vi "2진파일 읽기_쓰기.vi"() -> ()   [LabVIEW 2020]
uses:
  <vilib>/Utility/sysdir.llb/System Directory Type.ctl
panel:
  out "데이터":dbl[](array[numeric])
  in  "에러 입력":errorcluster
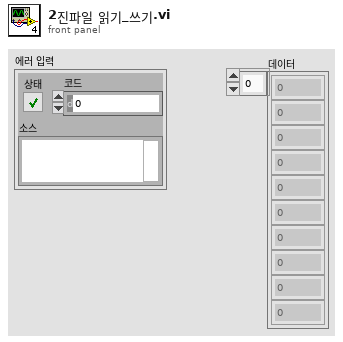
[diagram p1: front panel]
types:
  T1 = enum16{"open", "replace", "create", "open or create", "replace or create", "replace or create with confirmation"}
  T2 = typedef "System Directory Type.ctl" = i32
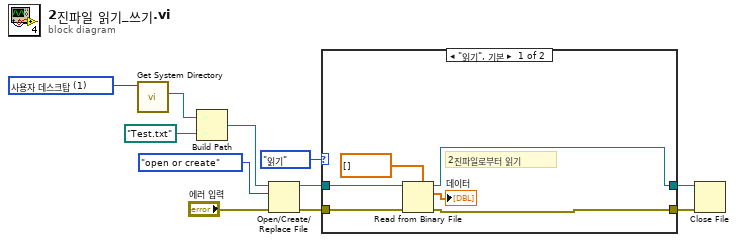
[diagram p0: block diagram]
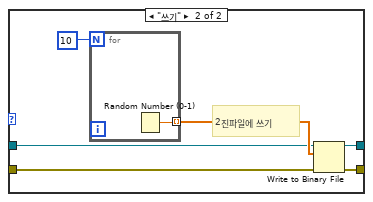
[diagram p2: hidden frame]
diagram:
  w10 = T2 1 items=["사용자 홈"=0, "사용자 데스크탑"=1, "사용자 문서"=2, "사용자 어플리케이션 데이터"=3, "사용자 환경"=4, "사용자 임시"=5, "퍼블릭 문서"=6, "퍼블릭 어플리케이션 데이터"=7, "퍼블릭 환경"=8, "퍼블릭 캐시"=13, "시스템 코어 라이브러리"=9, "시스템 설치된 라이브러리"=10, "어플리케이션 파일"=11, "부팅 볼륨 루트"=12] ("system directory type")
  n1 = call <vilib>:"Get System Directory.vi"("system directory type"=w10) -> ("system directory"=w9:path)  [unwired: 10 in]
  n2 = Build Path(base path=w9, name or relative path=path "Test.txt" ("이름 또는 상대 경로")) -> (appended path=w7:path)
  n3 = Open/Create/Replace File(file path (use dialog)=w7, error in="에러 입력", operation (0:open)=T1."open or create" ("동작(0:open)")) -> (refnum out=w4:refnum<file>, error out=w1:errorcluster)  [unwired: 3 in, 1 out]
  n4 = case shown="\"읽기\", 기본" enum16{"쓰기", "읽기"}."읽기" {
    tunnel: w4 -> [w15 w21]
    tunnel: [w14 w20] -> w3
    tunnel: [w13 w19] -> w2
    tunnel: w1 -> [w12 w18]
    frame "읽기", Default {
      # "2진파일로부터 읽기"
      n5 = Read from Binary File(5:dbl[] [], 8:w12, 11:w15) -> (0:w13:errorcluster, 2:→"데이터":dbl[], 3:w14:refnum<file>)  [unwired: 3 in, 1 out]
    }
    frame "쓰기" {
      # "2진파일에 쓰기"
      n6 = for {
        N: 10 -> [_]
        tunnel: [w24] -> w22 mode=indexing
        n7 = Random Number (0-1)() -> (number: 0 to 1=w24:dbl)
      }
      n8 = Write to Binary File(file (use dialog)=w21, data=w22, error in=w18) -> (refnum out=w20:refnum<file>, error out=w19:errorcluster)  [unwired: 3 in, 1 out]
    }
  }
  n9 = Close File(refnum=w3, error in=w2) -> ()  [unwired: 2 out]
